vi "start Report1.0 (SubVI).vi"(8 "error in (no error)":errorcluster, 11 "Serial Number":string) -> (0 "error out":errorcluster, 3 "Byte Stream File out":refnum<file>)   [LabVIEW 2013]
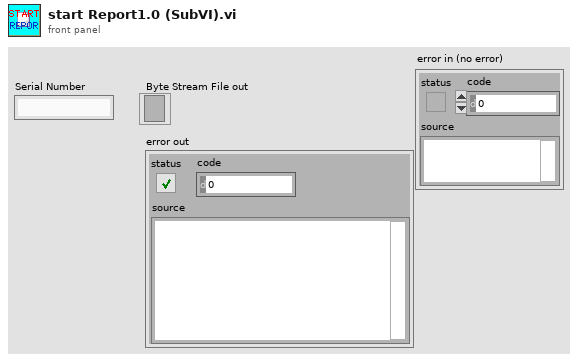
[diagram p1: front panel]
types:
  T1 = enum16{"open", "replace", "create", "open or create", "replace or create", "replace or create with confirmation"}
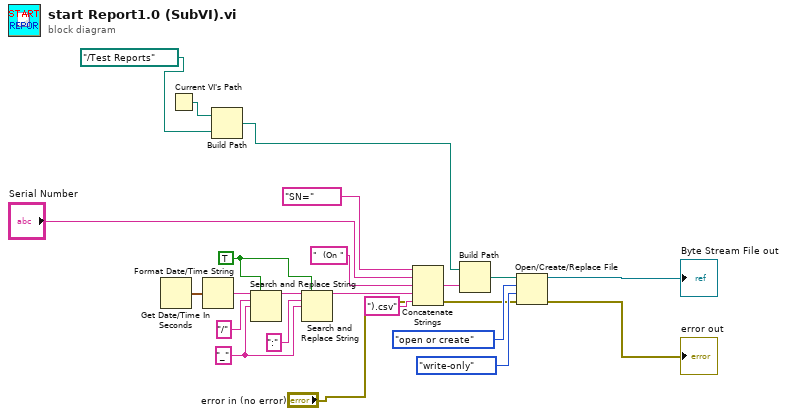
[diagram p0: block diagram]
diagram:
  w17 = TRUE ("replace all? (F)")
  w16 = "_"
  n1 = Get Date/Time In Seconds() -> (seconds since 1Jan1904=w11:timestamp)
  n2 = Current VI's Path() -> (path=w3:path)
  n3 = Format Date/Time String(seconds (now)=w11) -> (date/time string=w12:string)  [unwired: 2 in]
  n4 = Build Path(base path=w3, name or relative path=path "../Test Reports") -> (appended path=w2:path)
  n5 = Search and Replace String(replace all?=w17, input string=w12, search string="/", replace string=w16) -> (result string=w14:string)  [unwired: 4 in, 3 out]
  n6 = Search and Replace String(replace all?=w17, input string=w14, search string=":", replace string=w16) -> (result string=w22:string)  [unwired: 4 in, 3 out]
  n7 = Concatenate Strings("SN=", "Serial Number", "  (On ", w22, ").csv") -> (w10:string)
  n8 = Build Path(base path=w2, name or relative path=w10) -> (appended path=w5:path)
  n9 = Open/Create/Replace File(file path (use dialog)=w5, error in="error in (no error)", operation (0:open)=T1."open or create", access (0:read/write)=enum16{"read/write", "read-only", "write-only"}."write-only") -> (refnum out=→"Byte Stream File out":refnum<file>, error out=→"error out":errorcluster)  [unwired: 3 out]
